vi "GetCaptorData.vi"(6 "Graph in":cluster{dbl[], dbl[]}, 7 "Index":i32=250, 8 "error in":errorcluster, 9 "Length":i32=250, 11 "ON":bool) -> (0 "error out":errorcluster, 2 "Values":cluster{dbl[], dbl[]})   [LabVIEW 2012]
uses:
  GlobalVariables/HardwarePresent.vi
  GlobalVariables/CalibrationState.vi
  GlobalVariables/Samples.vi
  GlobalVariables/CurrentPressure.vi
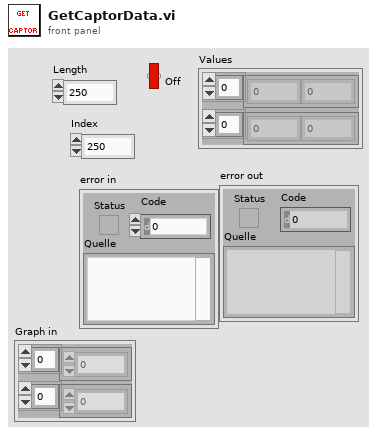
[diagram p1: front panel]
types:
  T1 = cluster{"CalibrationDone":bool, "CalibrationStep":u32, "Constante":dbl[], "Gain":dbl[]}
  T2 = cluster{"Pressure":cluster{"TimeSamples":dbl[], "PressureSamples":dbl[]}, "Flow":cluster{"TimeSamples":dbl[], "FlowSamples":dbl[]}}
  T3 = cluster{"TimeSamples":dbl[], "FlowSamples":dbl[]}
  T4 = cluster{cluster{dbl[], dbl[]}, "Flow":cluster{"TimeSamples":dbl[], "FlowSamples":dbl[]}}
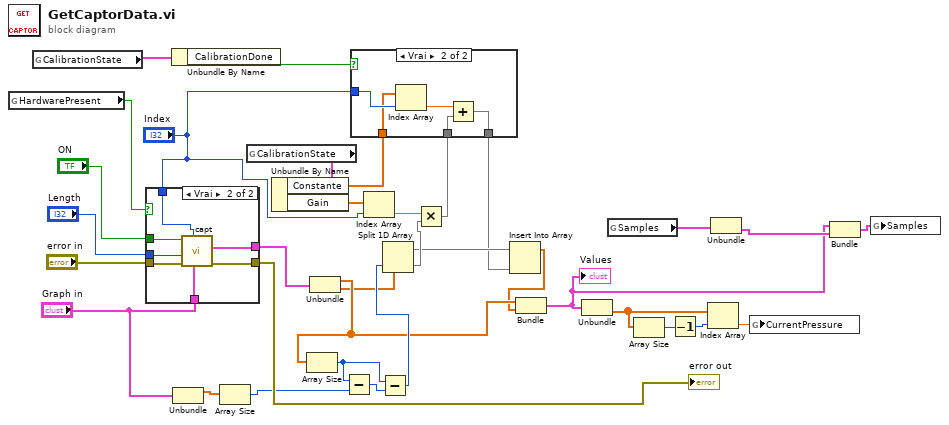
[diagram p0: block diagram]
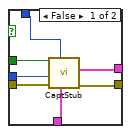
[diagram p3: hidden frame]
diagram:
  n1 = global read "HardwarePresent.vi" "HardwarePresent"() -> (w31:bool)
  n2 = global read "CalibrationState.vi" "CalibrationState"() -> (w29:T1)
  n3 = case shown="Vrai" w31 {
    tunnel: "Graph in" -> [w38 w48]
    tunnel: "error in" -> [w39 w45]
    tunnel: [w37 w46] -> w30
    tunnel: [w36 w47] -> w6
    tunnel: "Length" -> [w40 w44]
    tunnel: "ON" -> [w41 w43]
    tunnel: "Index" -> [w35 w42]
    frame False {
      n4 = call "CaptStub.vi"("Graph in"=w38, "Index"=w35, "error in"=w39, "Length"=w40, "ON"=w41) -> ("error out"=w37:errorcluster, "Values"=w36:cluster{dbl[], dbl[]})  [unwired: 5 in]
    }
    frame True {
      n5 = call "capt.vi"("Graph in"=w48, "Index"=w42, "error in"=w45, "Length"=w44, "ON"=w43) -> ("error out"=w46:errorcluster, "Values"=w47:cluster{dbl[], dbl[]})  [unwired: 5 in]
    }
  }
  "error out" <- w30
  n6 = Unbundle By Name(w29) -> ("CalibrationDone"=w28:bool)
  n7 = Unbundle("Graph in") -> (w21:dbl[])  [unwired: 1 out]
  n8 = Array Size(array=w21) -> (size(s)=w7:i32)
  n9 = global read "CalibrationState.vi" "CalibrationState"() -> (w9:T1)
  n10 = Unbundle By Name(w9) -> ("Constante"=w8:dbl[], "Gain"=w4:dbl[])
  n11 = Unbundle(w6) -> (w13:dbl[], w12:dbl[])
  n12 = Array Size(array=w13) -> (size(s)=w18:i32)
  n13 = Subtract(x=w18, y=w7) -> (x-y=w14:i32)
  n14 = Index Array(array=w4, index="Index") -> (element=w16:dbl)
  n15 = Subtract(x=w18, y=w14) -> (x-y=w15:i32)
  n16 = Split 1D Array(array=w12, index=w15) -> (first subarray=w10:dbl[], second subarray=w17:dbl[])
  n17 = Multiply(x=w16, y=w17) -> (x*y=w3:dbl[])
  n18 = case shown="Vrai" w28 {
    tunnel: "Index" -> [_ w54]
    tunnel: w8 -> [_ w53]
    tunnel: w3 -> [w49 w52]
    tunnel: [w49 w51] -> w2
    frame False {
    }
    frame True {
      n19 = Index Array(array=w53, index=w54) -> (element=w50:dbl)
      n20 = Add(x=w50, y=w52) -> (x+y=w51:dbl[])
    }
  }
  n21 = Insert Into Array(array=w10, new element=w2) -> (w11:dbl[])  [unwired: 1 in]
  n22 = Bundle(w13, w11) -> (w1:cluster{dbl[], dbl[]})  [unwired: 1 in]
  "Values" <- w1
  n23 = Unbundle(w1) -> (w25:dbl[])  [unwired: 1 out]
  n24 = global read "Samples.vi" "Samples"() -> (w23:T2)
  n25 = Array Size(array=w25) -> (size(s)=w19:i32)
  n26 = Decrement(x=w19) -> (x-1=w26:i32)
  n27 = Index Array(array=w25, index=w26) -> (element=w27:dbl)
  n28 = Unbundle(w23) -> ("Flow"=w22:T3)  [unwired: 1 out]
  n29 = global write "CurrentPressure.vi" "CurrentPressure"(w27) -> ()
  n30 = Bundle(w1, "Flow"=w22) -> (w24:T4)  [unwired: 1 in]
  n31 = global write "Samples.vi" "Samples"(w24) -> ()
